vi "Init_Test.vi"(8 "error in (no error)":errorcluster caption="entrée d'erreur (pas d'erreur)", 11 "Get_Voltage en entrée":refnum<class "Init_Power_Supply.lvclass">) -> (0 "error out":errorcluster caption="sortie d'erreur", 3 "Get_Voltage en sortie":refnum<class "Init_Power_Supply.lvclass">)   [LabVIEW 2020, in "Library Test.lvlib" / "Init_Power_Supply.lvclass"]
uses:
  Init_Power_Supply.lvclass
  C:/Users/ngarcin/OneDrive - Altyor/Standard TB/Class/Test/Test (Default)/Test (Default).lvclass
  Commun VI/TypeDef/Commande Test/Commande Value Type.ctl
  Commun VI/TypeDef/Commande Test/Commande Type Test.ctl
  Commun VI/TypeDef/Command Power_Supply/Parameter Power_Supply.ctl
  Power_Supply/Power_Supply (Default)/Power_Supply (Default).lvclass
  JSON API/JSON Value/Set from JSON string.vi
  JSON API/Variant JSON/Variant to JSON.vi
  JSON API/JSON Value/Get Item by name array.vi
  Test_Wtih_Instr/Test_With_Inst.lvclass
  Instrument/Instrument (Default)/Class Instrument (Default).lvclass
  JSON API/JSON Value/JSON Value.lvclass
  Init_Power_Supply.lvclass/Init_Power_Supply.ctl
  Commun VI/Library Commun.lvlib
  JSON API/Variant JSON/Variant JSON.lvlib
  JSON API/Get Polymorphic/JSON GetSet.lvlib
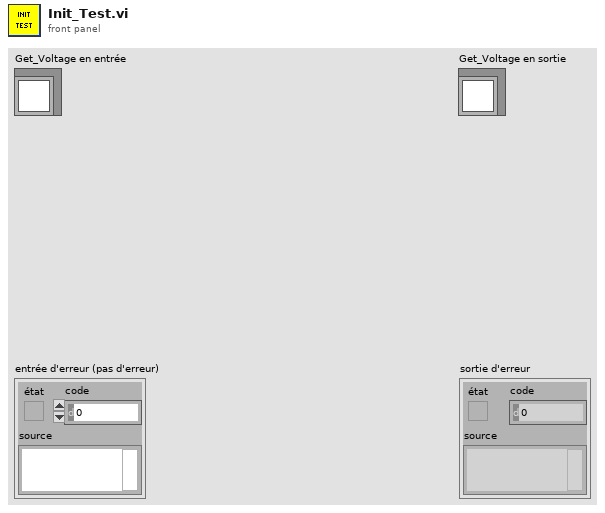
[diagram p1: front panel]
types:
  T1 = typedef "Library Commun.lvlib/Commande Type Test.ctl" = enum16{"Function", "Test", "Calculation"}
  T2 = typedef "Library Commun.lvlib/Commande Value Type.ctl" = enum16{"None", "String", "Number", "Timestamp", "Boolean", "Array"}
  T3 = typedef "Library Commun.lvlib/Parameter Power_Supply.ctl" = cluster{"Device_Addr":refnum<visa-resource-name>, "Current":dbl, "Channel":i32, "Voltage":dbl, " Class Power_Supply":refnum<class "Power_Supply (Default).lvclass">}
  T4 = cluster{"Current":dbl, "Channel":i32, "Voltage":dbl}
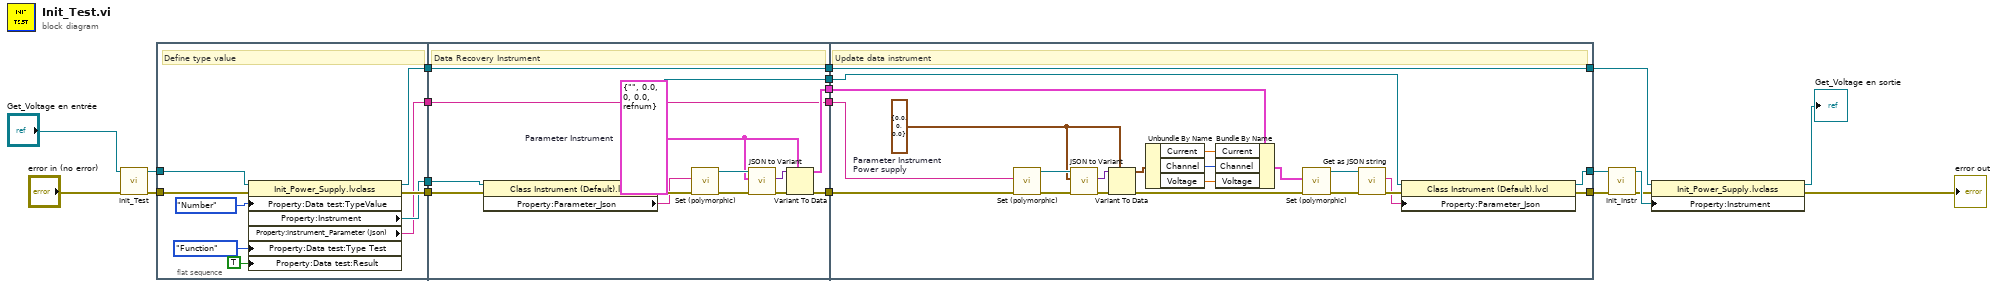
[diagram p0: block diagram]
diagram:
  n1 = call-parent "Init_Test.vi"("error in (no error)"="error in (no error)", "Test_With_Inst en entrée"="Get_Voltage en entrée") -> ("error out"=w12:errorcluster, "Test_With_Inst en sortie"=w13:refnum<class "Init_Power_Supply.lvclass">)  [unwired: 8 in]
  n2 = flat-sequence {
    tunnel: [w26] -> w15
    tunnel: [w25] -> w14
    tunnel: w13 -> [w29]
    tunnel: w12 -> [w28]
    tunnel: [w24] -> w10
    tunnel: [w23] -> w8
    tunnel: [w43] -> w18
    tunnel: [w34] -> w17
    tunnel: [w32] -> w16
    tunnel: w15 -> [w42]
    tunnel: w14 -> [w41]
    tunnel: [w33] -> w11
    tunnel: w10 -> [w33]
    tunnel: [w31] -> w9
    tunnel: w8 -> [w31]
    tunnel: w18 -> [w50]
    tunnel: w17 -> [w51]
    tunnel: w16 -> [w49]
    tunnel: [w47] -> w7
    tunnel: w11 -> [w48]
    tunnel: [w46] -> w6
    tunnel: w9 -> [w45]
    tunnel: [w45] -> w3
    frame #0 {
      # "Define type value"
      n3 = property class="Init_Power_Supply.lvclass"(reference=w29, error in=w28, "Property:Data test:TypeValue"=Commande_Value_Type."Number" ("TypeValue"), "Property:Data test:Type Test"=Commande_Type_Test."Function" ("Type Test"), "Property:Data test:Result"=TRUE ("Result")) -> (reference out=w23:refnum<class "Init_Power_Supply.lvclass">, error out=w26:errorcluster, "Property:Instrument"=w25:refnum<class "Class Instrument (Default).lvclass">, "Property:Instrument_Parameter (Json)"=w24:string)
    }
    frame #1 {
      w30 = T3 {"Device_Addr"="", "Current"=0.0, "Channel"=0, "Voltage"=0.0, " Class Power_Supply"=refnum}  # Parameter Instrument
      # "Data Recovery Instrument"
      n4 = property class="Class Instrument (Default).lvcl"(reference=w41, error in=w42) -> (reference out=w32:refnum<class "Class Instrument (Default).lvclass">, error out=w40:errorcluster, "Property:Parameter_Json"=w39:string)
      n5 = call-poly "Set (polymorphic).vi"("error in (no error)"=w40, "JSON stream"=w39) -> ("error out"=w37:errorcluster, "JSON Value out"=w35:refnum<class "JSON Value.lvclass">)  [unwired: 7 in, 1 out]
      n6 = call "JSON to Variant.vi"("error in (no error)"=w37, "Variant (Data Type)"=w30, "JSON Value"=w35) -> ("error out"=w36:errorcluster, "Variant out"=w38:variant)  [unwired: 7 in]
      n7 = Variant To Data(error in=w36, type=w30, Variant=w38) -> (data=w43:T3, error out=w34:errorcluster)
    }
    frame #2 {
      w44 = T4 {"Current"=0.0, "Channel"=0, "Voltage"=0.0}  # Parameter Instrument Power supply
      # "Update data instrument"
      n8 = call-poly "Set (polymorphic).vi"("error in (no error)"=w51, "JSON stream"=w48) -> ("error out"=w53:errorcluster, "JSON Value out"=w55:refnum<class "JSON Value.lvclass">)  [unwired: 7 in, 1 out]
      n9 = call "JSON to Variant.vi"("error in (no error)"=w53, "Variant (Data Type)"=w44, "JSON Value"=w55) -> ("error out"=w54:errorcluster, "Variant out"=w52:variant)  [unwired: 7 in]
      n10 = Variant To Data(error in=w54, type=w44, Variant=w52) -> (data=w56:T4, error out=w62:errorcluster)
      n11 = Unbundle By Name(w56) -> ("Current"=w57:dbl, "Channel"=w58:i32, "Voltage"=w59:dbl)
      n12 = Bundle By Name(cluster=w50, "Current"=w57, "Channel"=w58, "Voltage"=w59) -> (w63:T3)
      n13 = call-poly "Set (polymorphic).vi"("error in (no error)"=w62, "Variant"=w63) -> ("error out"=w60:errorcluster, "JSON Value out"=w61:refnum<class "JSON Value.lvclass">)  [unwired: 8 in]
      n14 = call "Get as JSON string.vi"("error in (no error)"=w60, "JSON Value in"=w61) -> ("error out"=w65:errorcluster, "<JSON>"=w64:string)  [unwired: 8 in]
      n15 = property class="Class Instrument (Default).lvcl"(reference=w49, error in=w65, "Property:Parameter_Json"=w64) -> (reference out=w46:refnum<class "Class Instrument (Default).lvclass">, error out=w47:errorcluster)
    }
  }
  n16 = call-dynamic "Init_Instr.vi"("error in (no error)"=w7, "Class Instrument (Default) en entrée"=w6) -> ("error out"=w2:errorcluster, "Class Instrument (Default) en sortie"=w5:refnum<class "Class Instrument (Default).lvclass">)  [unwired: 8 in]
  n17 = property class="Init_Power_Supply.lvclass"(reference=w3, error in=w2, "Property:Instrument"=w5) -> (reference out=→"Get_Voltage en sortie":refnum<class "Init_Power_Supply.lvclass">, error out=→"error out":errorcluster)
